vi "GetJoystickButton.vi"(11 "Array":bool[](array[boolean])) -> (0 "j3":bool, 1 "j2":bool, 2 "j1":bool, 3 "j0":bool)   [LabVIEW 2015]
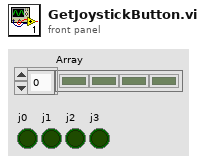
[diagram p1: front panel]
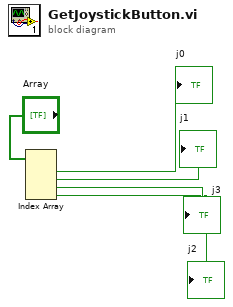
[diagram p0: block diagram]
diagram:
  n1 = Index Array(array="Array") -> (element #1=→"j0":bool, element #2=→"j1":bool, element #3=→"j3":bool, element #4=→"j2":bool)  [unwired: 4 in]
